vi "Write UI.vi"(10 "UI":refnum<class "Message Enqueuer.lvclass">, 11 "Cooler in":refnum<class "Cooler.lvclass">) -> (3 "Cooler out":refnum<class "Cooler.lvclass">)   [LabVIEW 2012, in "Cooler.lvlib" / "Cooler.lvclass"]
uses:
  Cooler.lvclass
  <vilib>/ActorFramework/Message Enqueuer/Message Enqueuer.lvclass
  Cooler.lvclass/Cooler.ctl
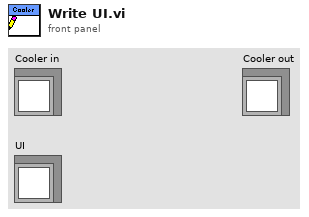
[diagram p1: front panel]
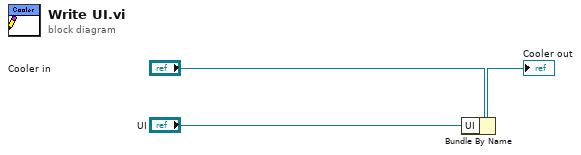
[diagram p0: block diagram]
diagram:
  n1 = Bundle By Name(cluster="Cooler in", "UI"="UI") -> (→"Cooler out":refnum<class "Cooler.lvclass">)
